vi "update_lc_tb_info.vi"(8 "cur_spnum":string, 9 "nx_spsta":string, 10 "nx_spren":string, 11 "lc_num":string) -> (2 "error":errorcluster caption="error out 4")   [LabVIEW 2017, in "Lib_code.lvlib"]
uses:
  Lib_code.lvlib
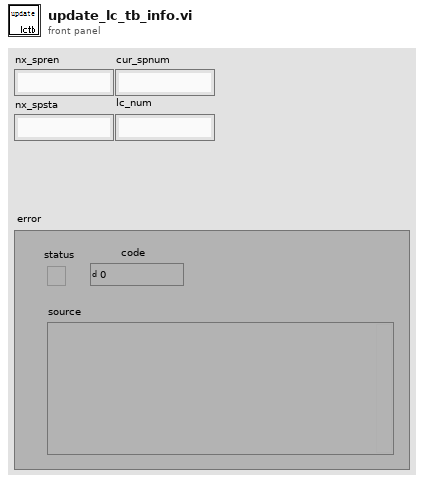
[diagram p1: front panel]
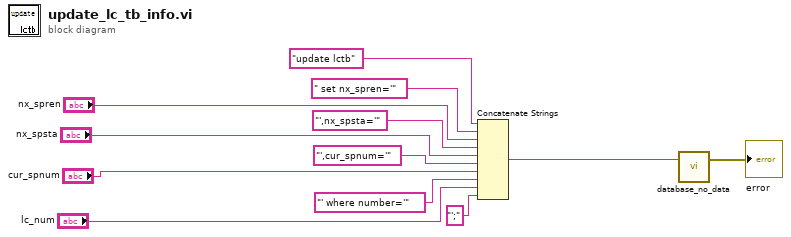
[diagram p0: block diagram]
diagram:
  n1 = Concatenate Strings("update lctb" ("Command Text"), " set nx_spren='" ("Command Text"), "nx_spren", "',nx_spsta='" ("字符串"), "nx_spsta", "',cur_spnum='" ("字符串"), "cur_spnum", "' where number='" ("字符串"), "lc_num", "';" ("字符串")) -> (w7:string)
  n2 = call "database_no_data.vi"("input"=w7) -> ("error"=→"error":errorcluster)  [unwired: 2 in]
